vi "EMV T7 Flow Detect.vi"(0 ".NET Refnum in":refnum<k24>, 1 "Detection Slope":dbl=0.2 format="%#_13g", 5 "ERD Data":T1, 7 "T7_DELTA_FLOW_THRESHOLD":dbl, 11 "error in (no error)":errorcluster) -> (4 ".NET Refnum out":refnum<k24>, 6 "Current T7 Temperatures":dbl[](array[numeric]), 8 "Flow Detect?":bool, 10 "T7 Slope Chart":dbl(graph), 15 "error out":errorcluster)   [LabVIEW 2020]
uses:
  C:/TechnologyLab/NI-2010/Drivers/GEA3 Toolkit/GEA3 DLL Source/GeaCommunication.dll
  GEA3 DLL Source/GeaCommunication.dll
  Type Definitions/GEA3 HEWH Mixing Valve.ctl
  Type Definitions/GEA3 HEWH ERD Data.ctl
panel:
  out "Unfiltered Flow Detect":bool
  out "End of Flow Detection?":bool
  in  "Abnormal Input Temperature":dbl=90.0
  out "T7 Acceleration Chart":dbl(graph)
  out "slope of slope":dbl
  out "slope standard deviation":dbl format="%0.2f"
  out "Slope History":dbl[](array[numeric])
  out "slope":dbl
  out "standard deviation":dbl format="%0.2f"
  in  "T7_DELTA_INDICATING_FLOW":dbl
  in  "Cold Water Supply Temperature":dbl
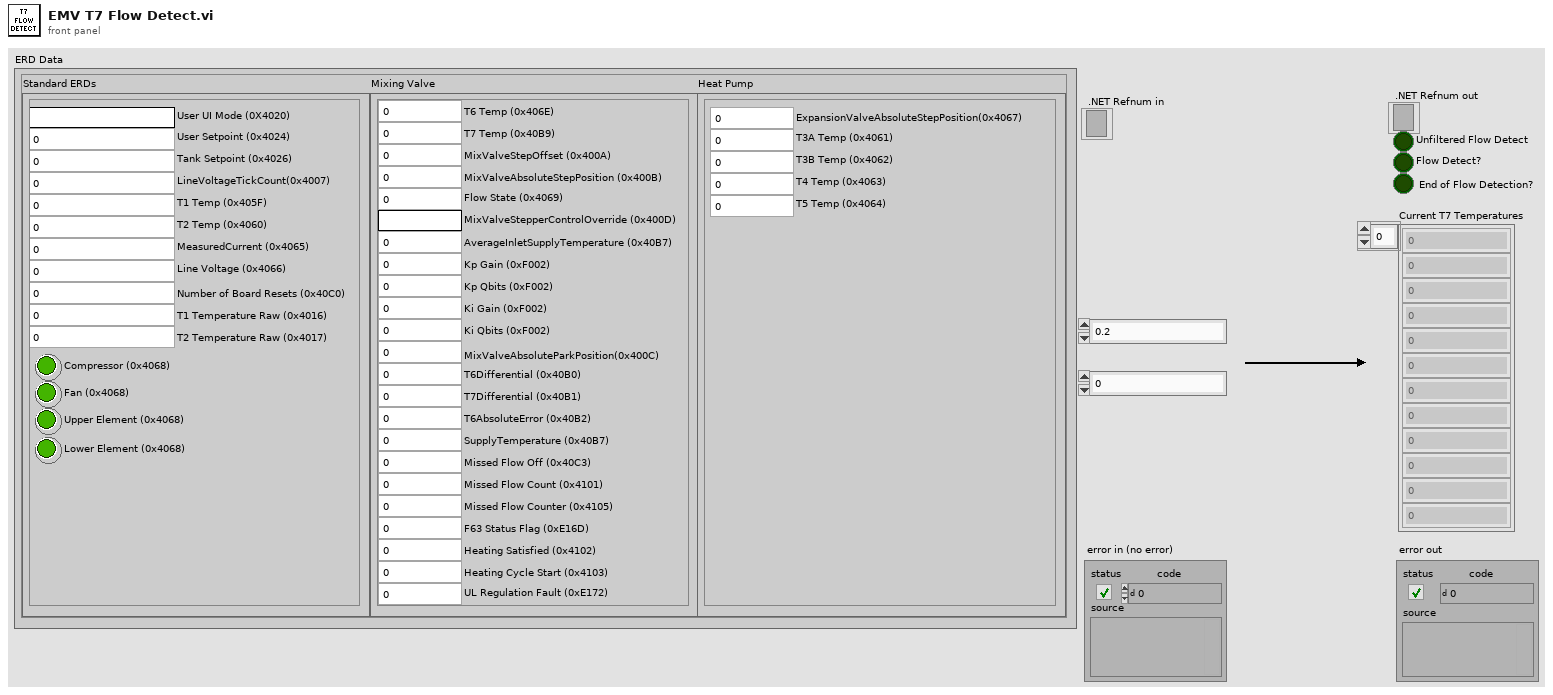
[diagram p1: front panel]
types:
  T1 = typedef "GEA3 HEWH ERD Data.ctl" = cluster{"Mixing Valve":T2, "Standard ERDs":cluster{"User UI Mode (0X4020)":string, "User Setpoint (0x4024)":u16, "Compressor (0x4068)":bool, "Lower Element (0x4068)":bool, "Upper Element (0x4068)":bool, "Fan (0x4068)":bool, "T1 Temp (0x405F)":dbl, "T2 Temp (0x4060)":dbl, "Line Voltage (0x4066)":dbl, "MeasuredCurrent (0x4065)":dbl, "LineVoltageTickCount(0x4007)":u16, "Number of Board Resets (0x40C0)":u16, "T1 Temperature Raw (0x4016)":u16, "T2 Temperature Raw (0x4017)":u16, "Tank Setpoint (0x4026)":u16}, "Heat Pump":cluster{"ExpansionValveAbsoluteStepPosition(0x4067)":i16, "T3A Temp (0x4061)":dbl, "T3B Temp (0x4062)":dbl, "T4 Temp (0x4063)":dbl, "T5 Temp (0x4064)":dbl}}
  T2 = typedef "GEA3 HEWH Mixing Valve.ctl" = cluster{"T7 Temp (0x40B9)":dbl, "MixValveStepOffset (0x400A)":i16, "MixValveAbsoluteStepPosition (0x400B)":i16, "Flow State (0x4069)":u8, "MixValveStepperControlOverride (0x400D)":string, "AverageInletSupplyTemperature (0x40B7)":dbl, "T6 Temp (0x406E)":dbl, "Kp Gain (0xF002)":u16, "Kp Qbits (0xF002)":u16, "Ki Gain (0xF002)":u16, "Ki Qbits (0xF002)":u16, "MixValveAbsoluteParkPosition(0x400C)":i16, "T7Differential (0x40B1)":dbl, "T6Differential (0x40B0)":dbl, "SupplyTemperature (0x40B7)":dbl, "Missed Flow Off (0x40C3)":u8, "T6AbsoluteError (0x40B2)":dbl, "Missed Flow Count (0x4101)":u16, "Missed Flow Counter (0x4105)":u16, "F63 Status Flag (0xE16D)":u16, "Heating Satisfied (0x4102)":u16, "Heating Cycle Start (0x4103)":u16, "UL Regulation Fault (0xE172)":u8}
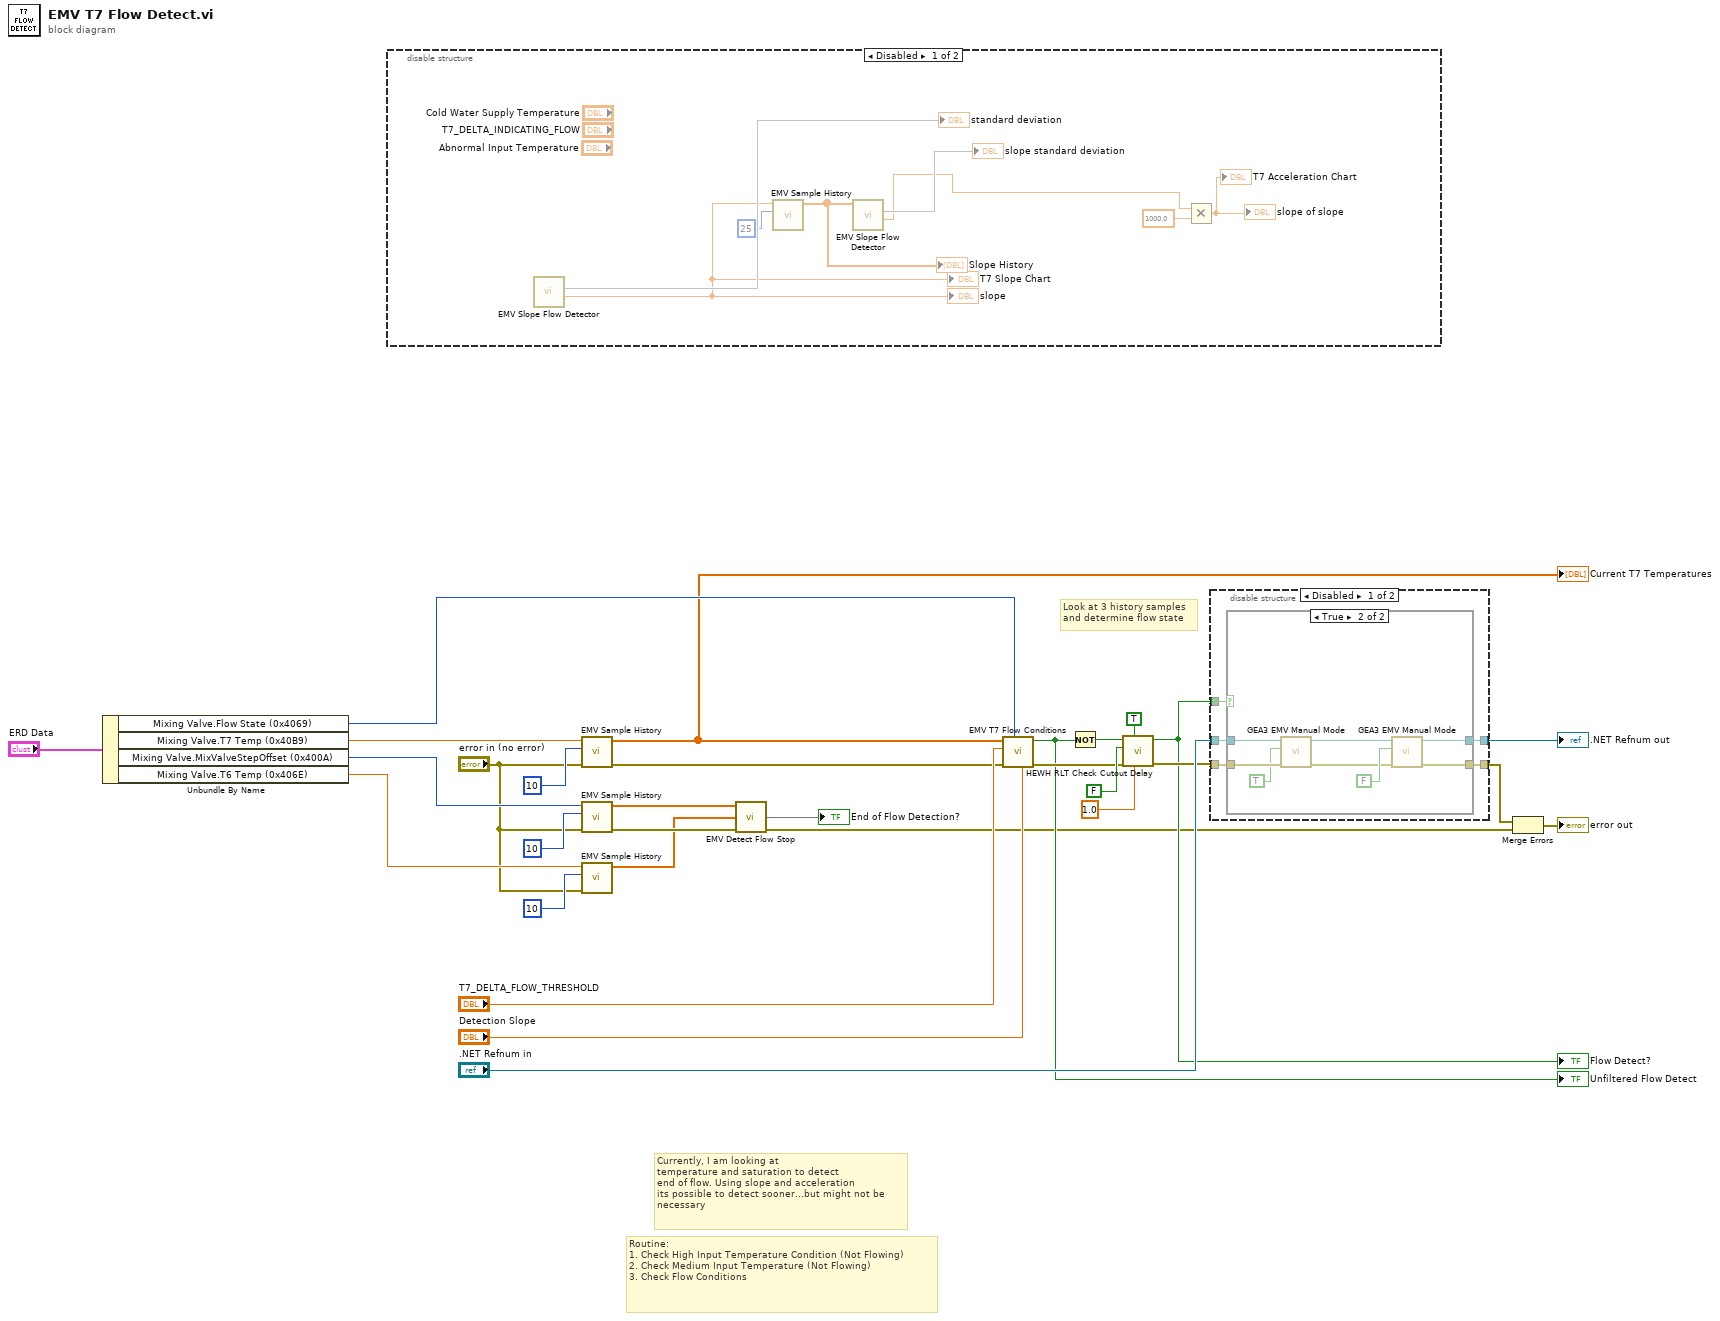
[diagram p0: block diagram]
diagram:
  # "Look at 3 history samples\nand determine flow state"
  # "Currently, I am looking at \ntemperature and saturation to detect\nend of flow. Using slope and acceleration\nits possible to detect sooner...but might not be \nnecessary"
  # "Routine:\n1. Check High Input Temperature Condition (Not Flowing)\n2. Check Medium Input Temperature (Not Flowing)\n3. Check Flow Conditions"
  n1 = Unbundle By Name("ERD Data") -> ("Mixing Valve.Flow State (0x4069)"=w22:u8, "Mixing Valve.T7 Temp (0x40B9)"=w23:dbl, "Mixing Valve.MixValveStepOffset (0x400A)"=w13:i16, "Mixing Valve.T6 Temp (0x406E)"=w3:dbl)
  n2 = disable-structure shown="Disabled" {
    frame Disabled {
      n3 = call "EMV Slope Flow Detector.vi"() -> ("slope"=w35:dbl, 2:→"standard deviation")  [unwired: 8 in, 2 out]
      "slope" <- w35
      "T7 Slope Chart" <- w35
      n4 = call "EMV Sample History.vi"("length"=25, "T6 Temp"=w35) -> ("T6 History"=w36:dbl[])  [unwired: 8 in, 1 out]
      "Slope History" <- w36
      n5 = call "EMV Slope Flow Detector.vi"("Current T6 Temperatures in"=w36) -> ("slope"=w32:dbl, 2:→"slope standard deviation")  [unwired: 7 in, 2 out]
      n6 = Multiply(x=w32, y=1000.0) -> (x*y=→"slope of slope" →"T7 Acceleration Chart":dbl)
    }
    frame Enabled {
    }
  }
  n7 = call "EMV Sample History.vi"("error in (no error)"="error in (no error)", "length"=10, "T6 Temp"=w23) -> ("error out"=w9:errorcluster, "T6 History"=w5:dbl[])  [unwired: 7 in]
  "Current T7 Temperatures" <- w5
  n8 = call "EMV Sample History.vi"("error in (no error)"="error in (no error)", "length"=10, "T6 Temp"=w13) -> ("error out"=w11:errorcluster, "T6 History"=w10:dbl[])  [unwired: 7 in]
  n9 = call "EMV Sample History.vi"("error in (no error)"="error in (no error)", "length"=10, "T6 Temp"=w3) -> ("T6 History"=w2:dbl[])  [unwired: 7 in, 1 out]
  n10 = call "EMV Detect Flow Stop.vi"("History Input"=w10, "T6"=w2, "error in (no error)"=w11) -> (8:→"End of Flow Detection?", "error out"=w7:errorcluster)  [unwired: 9 in, 2 out]
  n11 = call "EMV T7 Flow Conditions.vi"("Detection Slope"="Detection Slope", "Mixing Valve.Flow State (0x4009)"=w22, "error in (no error)"=w9, "T7_DELTA_FLOW_THRESHOLD"="T7_DELTA_FLOW_THRESHOLD", "T7 History"=w5) -> ("error out"=w18:errorcluster, "Flow Detect?"=w15:bool)  [unwired: 3 in, 2 out]
  "Unfiltered Flow Detect" <- w15
  n12 = Not(x=w15) -> (.not. x?=w14:bool)
  n13 = call "HEWH RLT Check Cutout Delay.vi"("Delay After Cutout (sec)"=1.0, "Use Cutout Delay"=TRUE, "Error In"=w18, "Start Draw"=FALSE, "Heat Source ON (1=ON)"=w14) -> ("Error Out"=w17:errorcluster, "Full Cutout?"=w16:bool)  [unwired: 5 in]
  "Flow Detect?" <- w16
  n14 = disable-structure shown="Disabled" {
    disable-tunnel: w16 -> [w43 _]
    disable-tunnel: [w42 w55] -> w8
    disable-tunnel: [w41 w54] -> w28
    disable-tunnel: w17 -> [w40 w55]
    disable-tunnel: ".NET Refnum in" -> [w39 w54]
    frame Disabled {
      n15 = case shown="True" w43 {
        tunnel: w40 -> [w45 w53]
        tunnel: [w45 w51] -> w42
        tunnel: w39 -> [w44 w52]
        tunnel: [w44 w50] -> w41
        frame False {
        }
        frame True {
          n16 = call "GEA3 EMV Manual Mode.vi"("error in (no error)"=w53, "Manual Mode?"=TRUE, ".NET Refnum in"=w52) -> ("error out"=w46:errorcluster, "GEA2 Reference Out"=w47:refnum<k24>)  [unwired: 7 in]
          n17 = call "GEA3 EMV Manual Mode.vi"("error in (no error)"=w46, "Manual Mode?"=FALSE, ".NET Refnum in"=w47) -> ("error out"=w51:errorcluster, "GEA2 Reference Out"=w50:refnum<k24>)  [unwired: 7 in]
        }
      }
    }
    frame Enabled {
    }
  }
  ".NET Refnum out" <- w28
  n18 = Merge Errors(w8, w7) -> (→"error out":errorcluster)
